vi "ROS_Topic_Close.vi"(0 "error in":errorcluster, 2 "ROS in":T1={"topic port"=0, "Node"="", "topic"="", "type"="", "node port"=0, "error "={"status"=FALSE, "code"=0, "source"=""}, "Direction"=enum."Node", "Update (ms)"=1, "queue size"=1}, 3 "node":string) -> (1 "error out":errorcluster)   [LabVIEW 2012]
doc: "Closes a topic. If no topic is defined, it will close all topics and all nodes."
uses:
  <userlib>/ROSforLV/ROS/Code/SubVIs/_ROSControl.ctl
  <userlib>/ROSforLV/ROS/Code/SubVIs/_ROSDirection.ctl
  <userlib>/ROSforLV/ROS/Code/_ROSDefinition.vi
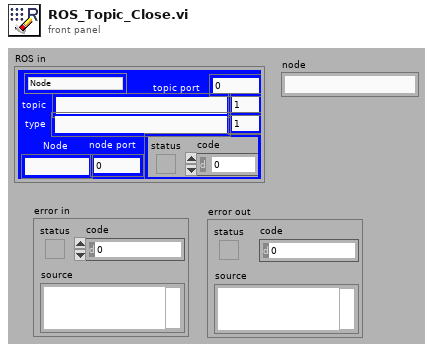
[diagram p1: front panel]
types:
  T1 = typedef "_ROSControl.ctl" = cluster{"topic port":u16, "Node":string, "topic":string, "type":string, "node port":u16, "error ":errorcluster, "Direction":T2, "Update (ms)":u16, "queue size":u16}
  T2 = typedef "_ROSDirection.ctl" = enum16{"Node", "Publisher", "Subscriber", "Service Client"}
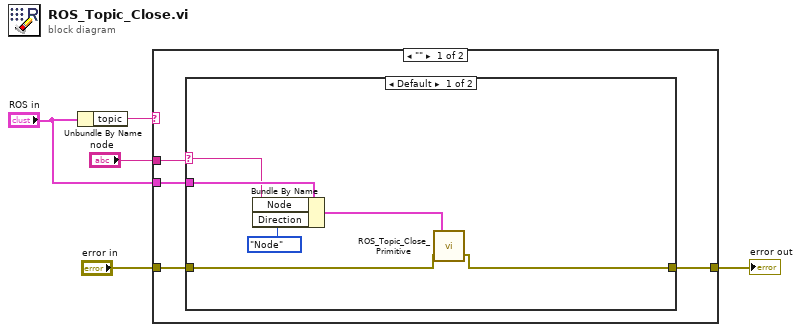
[diagram p0: block diagram]
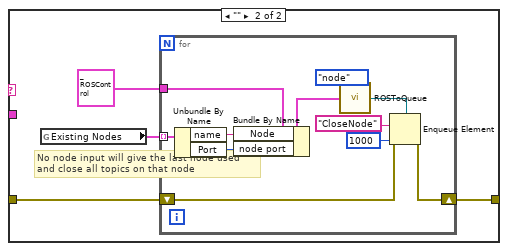
[diagram p2: hidden frame]
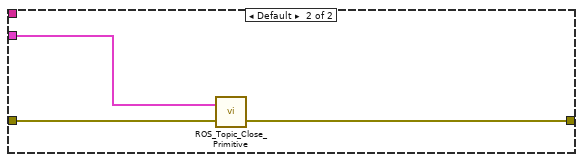
[diagram p3: hidden frame]
diagram:
  n1 = Unbundle By Name("ROS in") -> ("topic"=w2:string)
  n2 = case shown="\"\"" w2 {
    tunnel: "error in" -> [w9 w33]
    tunnel: "ROS in" -> [w6 w32]
    tunnel: [w8 w31] -> w3
    tunnel: "node" -> [w7 _]
    frame "" {
      n3 = case shown="Default" w7 {
        selector: w7 -> [w14 _]
        tunnel: w9 -> [w11 w17]
        tunnel: [w10 w16] -> w8
        tunnel: w6 -> [w15 _]
        frame Default {
          n4 = Bundle By Name(cluster=w15, "Node"=w14, "Direction"=_ROSDirection."Node") -> (w12:T1)
          n5 = call <userlib>:"ROS_Topic_Close_Primitive.vi"("error in"=w11, "ROS in"=w12) -> ("error out"=w10:errorcluster)  [unwired: 1 in]
        }
        frame "" {
          # "No node input will give the last node used\nand close all topics on that node"
          n6 = global read "_ROSDefinition.vi" "Existing Nodes"() -> (w18:cluster{"name":string, "Port":u16}[])
          n7 = for {
            tunnel: T1 {"topic port"=0, "Node"="", "topic"="", "type"="", "node port"=0, "error "={"status"=FALSE, "code"=0, "source"=""}, "Direction"=enum."Node", "Update (ms)"=1, "queue size"=1} ("ROS") -> [w26]
            tunnel: w18 -> [w24] mode=indexing
            shift-right: [w20] -> w16
            shift-left: w17 -> [w21]
            n8 = Unbundle By Name(w24) -> ("name"=w23:string, "Port"=w22:u16)
            n9 = Bundle By Name(cluster=w26, "Node"=w23, "node port"=w22) -> (w25:T1)
            n10 = call <userlib>:"ROSToQueue.vi"("ROS"=w25, "Name"=enum16{"topic", "node"}."node") -> ("queue"=w29:refnum<queue>)  [unwired: 2 in, 1 out]
            n11 = Enqueue Element(queue=w29, element="CloseNode" ("format string"), timeout in ms (-1)=1000, error in (no error)=w21) -> (error out=w20:errorcluster)  [unwired: 2 out]
          }
        }
      }
    }
    frame Default {
      n12 = call <userlib>:"ROS_Topic_Close_Primitive.vi"("error in"=w33, "ROS in"=w32) -> ("error out"=w31:errorcluster)  [unwired: 1 in]
    }
  }
  "error out" <- w3
